vi "RW Rem IO Slaves.vi"(7 "R/W Case":T10, 8 "error in (no error)":errorcluster, 10 "Async in":T9, 11 "REM IO EtherCAT Slave In":T1 {"I/O Output Data"."BD Refs"."Data Reference" format="%.0x"; "I/O Input Data"."BD Refs"."Data Reference" format="%.0x"; "I/O Output Vars"."VS ref" format="%.0x"; "I/O Imput Vars"."VS ref" format="%.0x"; "VS ref" format="%.0x"}) -> (0 "error out":errorcluster, 2 "Async out":T9, 3 "REM IO EtherCAT Slave Out":T1 {"I/O Output Data"."BD Refs"."Data Reference" format="%.0x"; "I/O Input Data"."BD Refs"."Data Reference" format="%.0x"; "I/O Output Vars"."VS ref" format="%.0x"; "I/O Imput Vars"."VS ref" format="%.0x"; "VS ref" format="%.0x"})   [LabVIEW 2016, in "Scan Engine Custom Device.lvlib"]
uses:
  Scan Engine Custom Device.lvlib
  Type Defs/RW Case.ctl
  Type Defs/Async Data.ctl
  Type Defs/Async Status.ctl
  Type Defs/Async State.ctl
  Type Defs/Async Command.ctl
  Type Defs/REM IO ECAT Slave Data Cluster.ctl
  <vilib>/NI Veristand/Custom Device API/Custom Device Item Ref.ctl
  Type Defs/REM IO ECAT Slave IOV Cluster.ctl
  Type Defs/UDV Data Type.ctl
  Type Defs/Input Data.ctl
  <vilib>/NI Veristand/Custom Device API/Block Data Reference.ctl
  <vilib>/NI Veristand/Custom Device API/Data Reference.ctl
  Type Defs/Output Data.ctl
  Scanned Read - UDV.vi
  <vilib>/NI Veristand/Custom Device API/NI VeriStand - Set Channel Values by Block Data Reference.vi
  Scanned Write - UDV.vi
  <vilib>/NI Veristand/Custom Device API/NI VeriStand - Get Channel Values by Block Data Reference.vi
  <vilib>/NI Veristand/Custom Device API/Global Data Refs.vi
  <vilib>/NI Veristand/Custom Device API/Custom Device API.lvlib
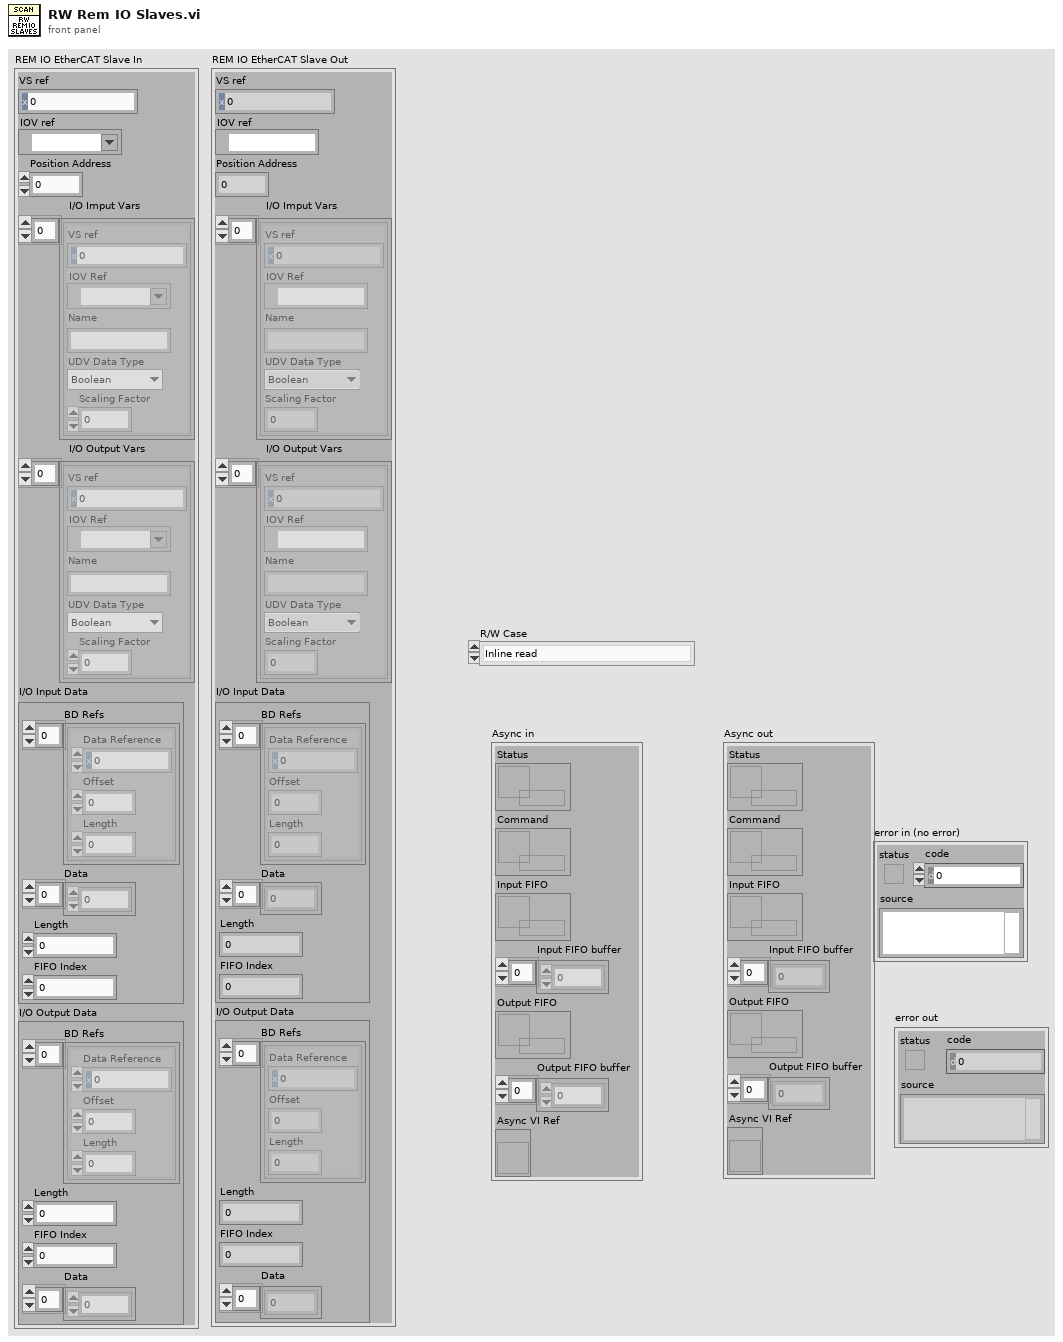
[diagram p1: front panel]
types:
  T1 = typedef "Scan Engine Custom Device.lvlib/REM IO ECAT Slave Data Cluster.ctl" = cluster{"VS ref":T2, "IOV ref":refnum<k21>, "Position Address":u16, "I/O Imput Vars ":T3[], "I/O Output Vars":T3[], "I/O Input Data":T5, "I/O Output Data":T8}
  T2 = typedef "Custom Device API.lvlib/Custom Device Item Ref.ctl" = u64
  T3 = typedef "Scan Engine Custom Device.lvlib/REM IO ECAT Slave IOV Cluster.ctl" = cluster{"VS ref":T2, "IOV Ref":refnum<k21>, "Name":string, "UDV Data Type":T4, "Scaling Factor":dbl}
  T4 = typedef "Scan Engine Custom Device.lvlib/UDV Data Type.ctl" = enum16{"Boolean", "Fixed Point", "Int8", "Int16", "Int32", "Int64", "U32 Bit Field", "UInt8", "UInt16", "UInt32", "UInt64", "Other"}
  T5 = typedef "Scan Engine Custom Device.lvlib/Input Data.ctl" = cluster{"BD Refs":T6[], "Data":dbl[], "Length":i32, "FIFO Index":i32}
  T6 = typedef "Custom Device API.lvlib/Block Data Reference.ctl" = cluster{"Data Reference":T7, "Offset":u64, "Length":u64}
  T7 = typedef "Custom Device API.lvlib/Data Reference.ctl" = i32
  T8 = typedef "Scan Engine Custom Device.lvlib/Output Data.ctl" = cluster{"BD Refs":T6[], "Length":i32, "FIFO Index":i32, "Data":dbl[]}
  T9 = typedef "Scan Engine Custom Device.lvlib/Async Data.ctl" = cluster{"Status":refnum<queue>, "Command":refnum<queue>, "Input FIFO":refnum<k33>, "Input FIFO buffer":dbl[], "Output FIFO":refnum<k33>, "Output FIFO buffer":dbl[], "Async VI Ref":refnum<vi>}
  T10 = typedef "Scan Engine Custom Device.lvlib/RW Case.ctl" = enum16{"Inline read", "Inline write", "Async - Inline loop read", "Async - Inline loop write", "Async loop (read/write)"}
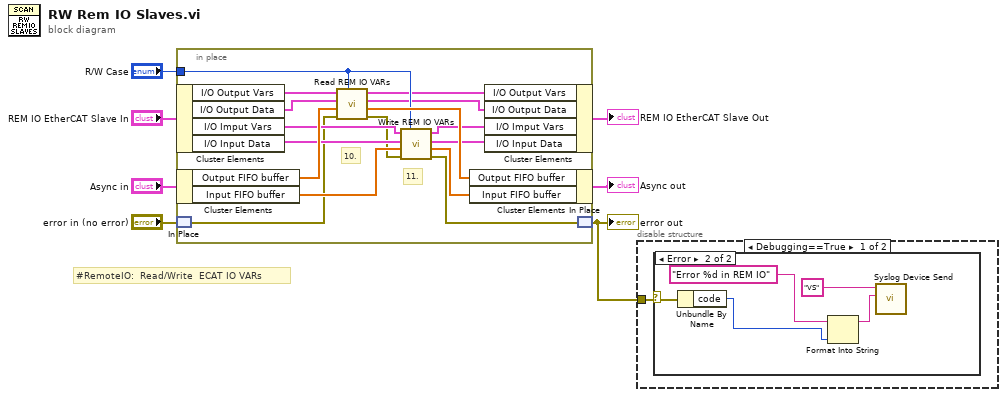
[diagram p0: block diagram]
diagram:
  # "#RemoteIO:  Read/Write  ECAT IO VARs"
  n1 = in-place {
    in-place-border: "R/W Case" -> [w19]
    # "11."
    # "10."
    n2 = in-place-cluster #1("REM IO EtherCAT Slave In") -> ("I/O Output Vars"=w18:T3[], "I/O Output Data"=w14:T8, "I/O Imput Vars"=w17:T3[], "I/O Input Data"=w12:T5)
    n3 = in-place-cluster #2("Async in") -> ("Output FIFO buffer"=w22:dbl[], "Input FIFO buffer"=w21:dbl[])
    n4 = in-place-match #3("error in (no error)") -> (w10:errorcluster)
    n5 = call "Read REM IO VARs.vi"("R/W Case"=w19, "error in (no error)"=w10, "Output FIFO buffer in"=w22, "I/O Output Data In"=w14, "I/O Output Vars in"=w18) -> ("error out"=w9:errorcluster, "Output FIFO buffer out"=w23:dbl[], "I/O Output Data Out"=w13:T8, "I/O Output Vars out"=w16:T3[])  [unwired: 3 in]
    n6 = call "Write REM IO VARs.vi"("R/W Case"=w19, "error in (no error)"=w9, "Input FIFO buffer in"=w21, "I/O Input Data In"=w12, "I/O Imput Vars in"=w17) -> ("error out"=w8:errorcluster, "Input FIFO buffer out"=w20:dbl[], "I/O Input Data Out"=w11:T5, "I/O Imput Vars out"=w15:T3[])  [unwired: 3 in]
    n7 = in-place-cluster #2("Output FIFO buffer"=w23, "Input FIFO buffer"=w20) -> (→"Async out":T9)
    n8 = in-place-cluster #1("I/O Output Vars"=w16, "I/O Output Data"=w13, "I/O Imput Vars"=w15, "I/O Input Data"=w11) -> (→"REM IO EtherCAT Slave Out":T1)
    n9 = in-place-match #3(w8) -> (w1:errorcluster)
  }
  "error out" <- w1
  n10 = disable-structure shown="Debugging==True" {
    disable-tunnel: w1 -> [w24 _]
    frame condition #0 (active) {
      n11 = case shown="Error" w24 {
        selector: w24 -> [_ w26]
        frame No Error {
        }
        frame Error {
          n12 = Unbundle By Name(w26) -> ("code"=w25:i32)
          n13 = Format Into String(format string="Error %d in REM IO", w25) -> (resulting string=w27:string)  [unwired: 2 in, 1 out]
          n14 = call <vilib>:"Syslog Device Send.vi"("Message Content"=w27, "Message Tag"="VS") -> ()  [unwired: 8 in, 2 out]
        }
      }
    }
    frame condition #1 {
    }
  }
